vi "IsEmpty.vi"(8 "error in (no error)":errorcluster, 11 "LinkedList in":refnum<class "LinkedList.lvclass">) -> (0 "error out":errorcluster, 1 "empty":bool, 3 "LinkedList out":refnum<class "LinkedList.lvclass">)   [LabVIEW 2014, in "LinkedList.lvlib" / "LinkedList.lvclass"]
doc: "Checks to see is the Linked List is empty."
uses:
  <userlib>/AdvancedDataStructures/ClassBased/LinkedList/LinkedList.lvclass
  <userlib>/AdvancedDataStructures/ClassBased/LinkedList/LinkedList.lvclass/LinkedList.ctl
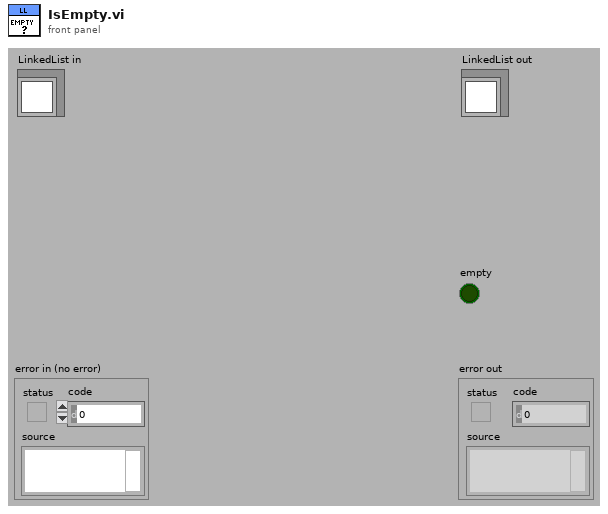
[diagram p1: front panel]
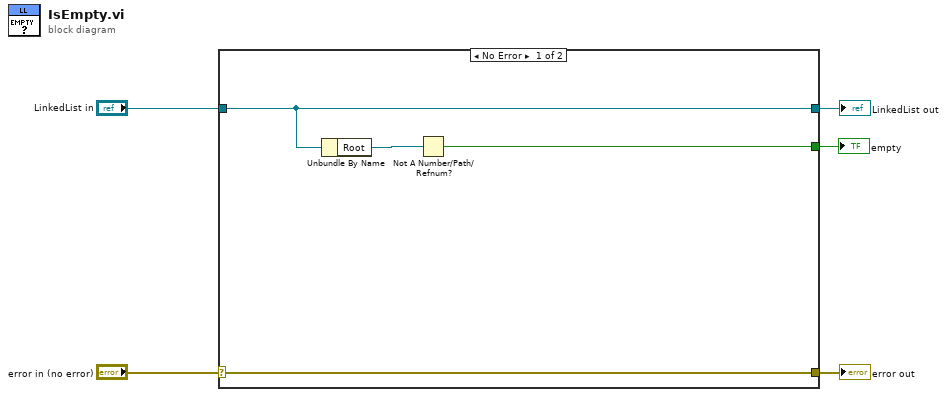
[diagram p0: block diagram]
diagram:
  n1 = case shown="No Error" "error in (no error)" {
    selector: "error in (no error)" -> [w9 w11]
    tunnel: [w9 w11] -> w4
    tunnel: [w8 w10] -> w2
    tunnel: "LinkedList in" -> [w8 w10]
    tunnel: [w6 _] -> w1
    frame No Error {
      n2 = Unbundle By Name(w8) -> ("Root"=w7:refnum<data-value>)
      n3 = Not A Number/Path/Refnum?(number/path/refnum=w7) -> (NaN/Path/Refnum?=w6:bool)
    }
    frame Error {
    }
  }
  "error out" <- w4
  "LinkedList out" <- w2
  "empty" <- w1
